vi "Prober_MoveToHome.vi"(8 "error in (no error)":errorcluster, 11 "AlessiRel6100 in":refnum<class "AlessiRel6100.lvclass">) -> (0 "error out":errorcluster, 3 "AlessiRel6100 out":refnum<class "AlessiRel6100.lvclass">)   [LabVIEW 2019, in "AlessiRel6100.lvclass"]
uses:
  AlessiRel6100.lvclass
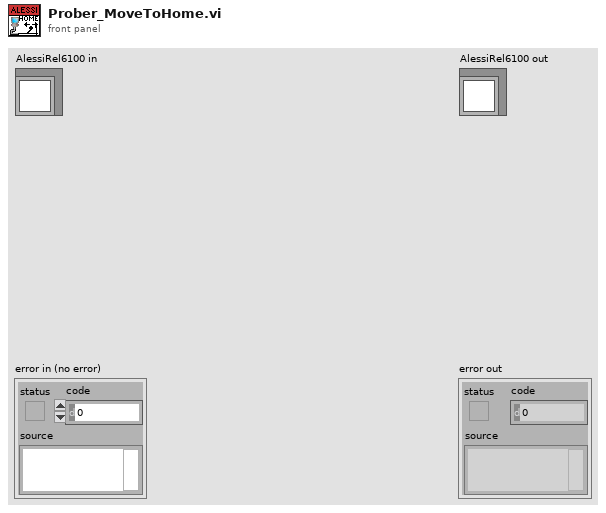
[diagram p1: front panel]
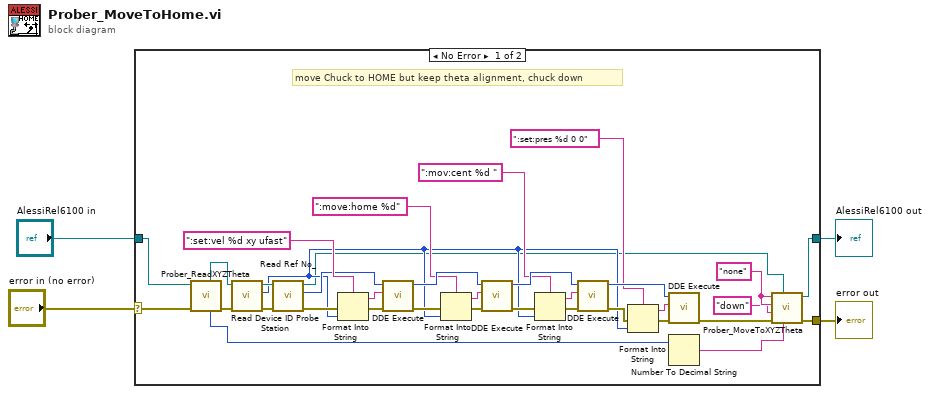
[diagram p0: block diagram]
diagram:
  n1 = case shown="No Error" "error in (no error)" {
    selector: "error in (no error)" -> [w5 w40]
    tunnel: "AlessiRel6100 in" -> [w27 w41]
    tunnel: [w29 w41] -> w2
    tunnel: [w28 w40] -> w1
    frame No Error {
      w37 = "none"
      # "move Chuck to HOME but keep theta alignment, chuck down"
      n2 = call-dynamic "Prober_ReadXYZTheta.vi"("error in (no error)"=w5, "AlessiRel6100 in"=w27) -> ("error out"=w23:errorcluster, "Theta location [mdeg]"=w26:i32, "AlessiRel6100 out"=w25:refnum<class "AlessiRel6100.lvclass">)  [unwired: 4 in, 3 out]
      n3 = call-dynamic "Read Device ID Probe Station.vi"("error in (no error)"=w23, "AlessiRel6100 in"=w25) -> ("error out"=w22:errorcluster, "Device ID Probe Station"=w8:u32, "AlessiRel6100 out"=w24:refnum<class "AlessiRel6100.lvclass">)  [unwired: 7 in]
      n4 = call-dynamic "Read Ref No_.vi"("error in (no error)"=w22, "AlessiRel6100 in"=w24) -> ("error out"=w20:errorcluster, "Ref No."=w17:u32, "AlessiRel6100 out"=w7:refnum<class "AlessiRel6100.lvclass">)  [unwired: 7 in]
      n5 = Format Into String(format string=":set:vel %d xy ufast" ("command"), error in=w20, w8) -> (resulting string=w18:string, error out=w19:errorcluster)  [unwired: 1 in]
      n6 = call <vilib>:"DDE Execute.vi"("error in (no error)"=w19, "command"=w18, "conversation refnum in"=w17) -> ("error out"=w16:errorcluster, "conversation refnum out"=w36:u32)  [unwired: 5 in]
      n7 = Format Into String(format string=":move:home %d", error in=w16, w8) -> (resulting string=w35:string, error out=w15:errorcluster)  [unwired: 1 in]
      n8 = call <vilib>:"DDE Execute.vi"("error in (no error)"=w15, "command"=w35, "conversation refnum in"=w36) -> ("error out"=w14:errorcluster, "conversation refnum out"=w33:u32)  [unwired: 5 in]
      n9 = Format Into String(format string=":mov:cent %d " ("command"), error in=w14, w8) -> (resulting string=w32:string, error out=w13:errorcluster)  [unwired: 1 in]
      n10 = call <vilib>:"DDE Execute.vi"("error in (no error)"=w13, "command"=w32, "conversation refnum in"=w33) -> ("error out"=w11:errorcluster, "conversation refnum out"=w30:u32)  [unwired: 5 in]
      n11 = Format Into String(format string=":set:pres %d 0 0" ("command"), error in=w11, w8) -> (resulting string=w9:string, error out=w10:errorcluster)  [unwired: 1 in]
      n12 = call <vilib>:"DDE Execute.vi"("error in (no error)"=w10, "command"=w9, "conversation refnum in"=w30) -> ("error out"=w38:errorcluster)  [unwired: 5 in, 1 out]
      n13 = Number To Decimal String(number=w26) -> (decimal integer string=w39:string)  [unwired: 1 in]
      n14 = call-dynamic "Prober_MoveToXYZTheta.vi"("Theta location [mdeg]"=w39, "AlessiRel6100 in"=w7, "error in (no error)"=w38, "Z location [µm]"="down", "Y location [µm]"=w37, "X location [µm]"=w37) -> ("error out"=w28:errorcluster, "AlessiRel6100 out"=w29:refnum<class "AlessiRel6100.lvclass">)  [unwired: 3 in, 1 out]
    }
    frame Error {
    }
  }
  "error out" <- w1
  "AlessiRel6100 out" <- w2
